vi "PIM Handle Swept Plot Trace.vi"(4 "Hold?":bool, 6 "Clear Plot? (f)":bool, 9 "Sweep Leg":enum16{"F2Down", "F1Up"}(ring), 10 "IM Freq":dbl format="%.2f", 11 "IM Power":dbl format="%.2f") -> (2 "F2 Down Trace":cluster{"new array":dbl[], "new array":dbl[]} {"new array" format="%.2f"; "new array" format="%.2f"}, 3 "F1 Up Trace":cluster{"new array":dbl[], "new array":dbl[]} {"new array" format="%.2f"; "new array" format="%.2f"})   [LabVIEW 2011]
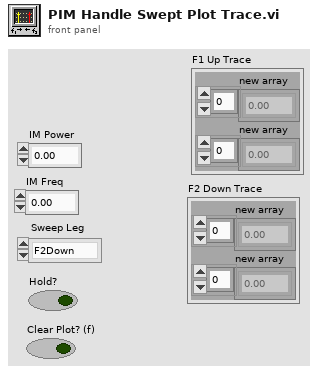
[diagram p1: front panel]
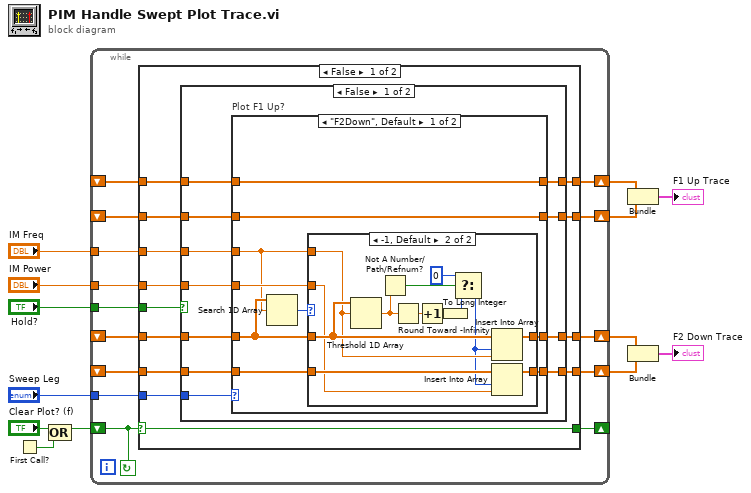
[diagram p0: block diagram]
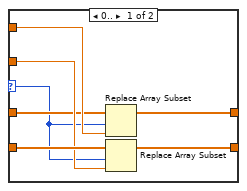
[diagram p2: hidden frame]
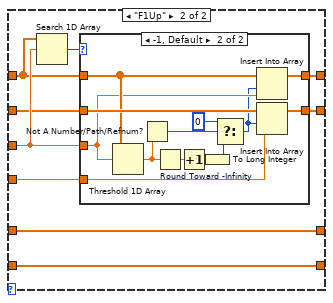
[diagram p3: hidden frame]
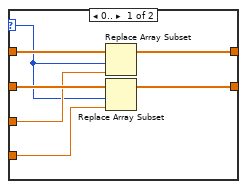
[diagram p4: hidden frame]
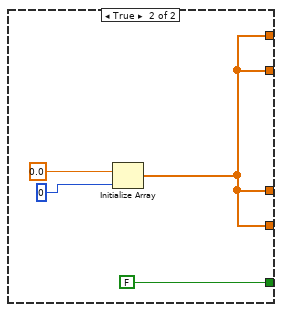
[diagram p6: hidden frame]
diagram:
  n1 = First Call?() -> (First Call?: T/F=w2:bool)
  n2 = Compound Arithmetic op=OR("Clear Plot? (f)", w2) -> (w1:bool)
  n3 = while {
    shift-right: [w25] -> w8
    shift-left: _ -> [w20]
    shift-right: [w24] -> w7
    shift-left: _ -> [w19]
    shift-right: [w27] -> w6
    shift-left: _ -> [w21]
    shift-right: [w26] -> w5
    shift-left: _ -> [w22]
    tunnel: "Sweep Leg" -> [w23]
    tunnel: "IM Freq" -> [w18]
    tunnel: "IM Power" -> [w17]
    shift-right: [w16] -> _
    shift-left: w1 -> [w14]
    tunnel: "Hold?" -> [w15]
    stop <- w14 continue-if-true
    n4 = case shown="False" w14 {
      selector: w14 -> [w30 _]
      tunnel: [w37 w116] -> w27
      tunnel: [w39 w116] -> w26
      tunnel: [w34 w116] -> w25
      tunnel: [w33 w116] -> w24
      tunnel: w23 -> [w28 _]
      tunnel: w22 -> [w40 _]
      tunnel: w21 -> [w38 _]
      tunnel: w20 -> [w36 _]
      tunnel: w19 -> [w35 _]
      tunnel: w18 -> [w32 _]
      tunnel: w17 -> [w31 _]
      tunnel: [w30 FALSE] -> w16
      tunnel: w15 -> [w29 _]
      frame False {
        n5 = case shown="False" w29 {
          tunnel: w40 -> [w51 w110]
          tunnel: [w50 w110] -> w39
          tunnel: w38 -> [w49 w111]
          tunnel: [w48 w111] -> w37
          tunnel: w36 -> [w47 w113]
          tunnel: w35 -> [w46 w112]
          tunnel: [w45 w113] -> w34
          tunnel: [w44 w112] -> w33
          tunnel: w32 -> [w43 _]
          tunnel: w31 -> [w42 _]
          tunnel: w28 -> [w41 _]
          frame False {
            n6 = case "Plot F1 Up?" shown="\"F2Down\", Default" w41 {
              tunnel: w46 -> [w60 w84]
              tunnel: [w60 w82] -> w44
              tunnel: w42 -> [w57 w86]
              tunnel: w51 -> [w59 w89]
              tunnel: [w58 w89] -> w50
              tunnel: w43 -> [w53 w87]
              tunnel: [w55 w83] -> w45
              tunnel: [w56 w88] -> w48
              tunnel: w49 -> [w54 w88]
              tunnel: w47 -> [w55 w85]
              frame "F2Down", Default {
                n7 = Search 1D Array(1D array=w54, element=w53) -> (index of element=w52:i32)  [unwired: 1 in]
                n8 = case shown="-1, Default" w52 {
                  selector: w52 -> [w61 _]
                  tunnel: w59 -> [w67 w78]
                  tunnel: [w66 w79] -> w58
                  tunnel: w57 -> [w65 w75]
                  tunnel: [w64 w77] -> w56
                  tunnel: w53 -> [w63 w76]
                  tunnel: w54 -> [w62 w80]
                  frame 0.. {
                    n9 = Replace Array Subset(array=w62, new element=w63, index=w61) -> (w64:dbl[])
                    n10 = Replace Array Subset(array=w67, new element=w65, index=w61) -> (w66:dbl[])
                  }
                  frame -1, Default {
                    n11 = Threshold 1D Array(2:w76, 3:w80) -> (0:w72:dbl)  [unwired: 1 in]
                    n12 = Not A Number/Path/Refnum?(number/path/refnum=w72) -> (NaN/Path/Refnum?=w71:bool)
                    n13 = Round Toward -Infinity(1:w72) -> (0:w74:dbl)
                    n14 = Increment(x=w74) -> (x+1=w73:dbl)
                    n15 = To Long Integer(number=w73) -> (32bit integer=w68:i32)
                    n16 = Select(t=0, s=w71, f=w68) -> (s? t:f=w69:i32)
                    n17 = Insert Into Array(array=w80, index=w69, new element=w76) -> (w77:dbl[])
                    n18 = Insert Into Array(array=w78, index=w69, new element=w75) -> (w79:dbl[])
                  }
                }
              }
              frame "F1Up" {
                n19 = Search 1D Array(1D array=w85, element=w87) -> (index of element=w81:i32)  [unwired: 1 in]
                n20 = case shown="-1, Default" w81 {
                  selector: w81 -> [w90 _]
                  tunnel: w84 -> [w96 w108]
                  tunnel: [w95 w109] -> w82
                  tunnel: w86 -> [w94 w106]
                  tunnel: [w93 w107] -> w83
                  tunnel: w87 -> [w92 w99]
                  tunnel: w85 -> [w91 w100]
                  frame 0.. {
                    n21 = Replace Array Subset(array=w91, new element=w92, index=w90) -> (w93:dbl[])
                    n22 = Replace Array Subset(array=w96, new element=w94, index=w90) -> (w95:dbl[])
                  }
                  frame -1, Default {
                    n23 = Threshold 1D Array(2:w99, 3:w100) -> (0:w103:dbl)  [unwired: 1 in]
                    n24 = Not A Number/Path/Refnum?(number/path/refnum=w103) -> (NaN/Path/Refnum?=w102:bool)
                    n25 = Round Toward -Infinity(1:w103) -> (0:w105:dbl)
                    n26 = Increment(x=w105) -> (x+1=w104:dbl)
                    n27 = To Long Integer(number=w104) -> (32bit integer=w101:i32)
                    n28 = Select(t=0, s=w102, f=w101) -> (s? t:f=w97:i32)
                    n29 = Insert Into Array(array=w100, index=w97, new element=w99) -> (w107:dbl[])
                    n30 = Insert Into Array(array=w108, index=w97, new element=w106) -> (w109:dbl[])
                  }
                }
              }
            }
          }
          frame True {
            # "Hold Sweep ... no plot updates"
          }
        }
      }
      frame True {
        n31 = Initialize Array(0.0, 0 ("Dimension Size")) -> (w116:dbl[])
      }
    }
  }
  n32 = Bundle(w8, w7) -> (→"F1 Up Trace":cluster{dbl[], dbl[]})  [unwired: 1 out]
  n33 = Bundle(w6, w5) -> (→"F2 Down Trace":cluster{dbl[], dbl[]})  [unwired: 1 out]
